vi "Noyito10ChannelADC_ManualPollingExample.vi"(8 "error in (no error)":errorcluster) -> (0 "error out":errorcluster, 1 "userMessage":string, 3 "readBuffer":string)   [LabVIEW 2020]
uses:
  <vilib>/Instr/_visa.llb/VISA Configure Serial Port (Instr).vi
panel:
  in  "Polling Speed":bool
  out "Num bytes":u32=115200
  in  "STOP POLLING":bool
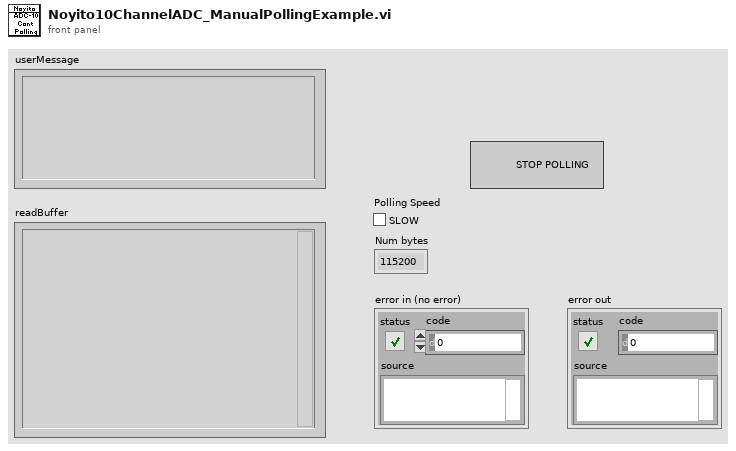
[diagram p1: front panel]
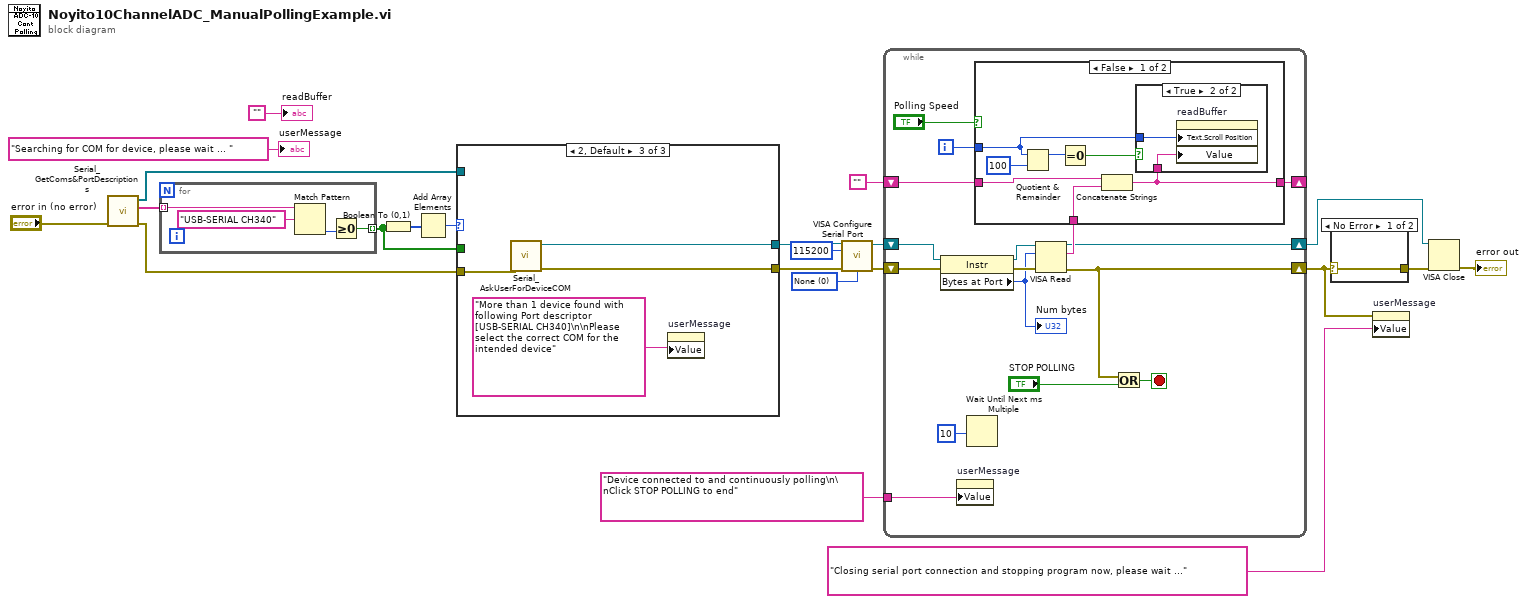
[diagram p0: block diagram]
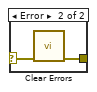
[diagram p2: hidden frame]
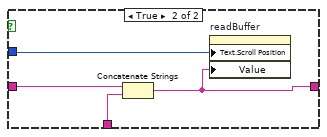
[diagram p4: hidden frame]
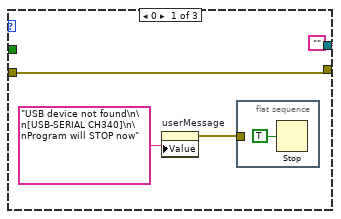
[diagram p5: hidden frame]
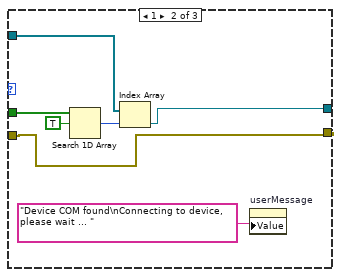
[diagram p6: hidden frame]
diagram:
  w11 = u16 0 items=["None", "XON/XOFF", "RTS/CTS", "XON/XOFF & RTS/CTS", "DTR/DSR", "XON/XOFF & DTR/DSR"] ("flow control (0:none)")
  n1 = call "Serial_GetComs&PortDescriptions.vi"("error in (no error)"="error in (no error)") -> ("error out"=w17:errorcluster, "WinsDescriptions"=w21:string[], "COMs"=w15:refnum<visa-resource-name>[])  [unwired: 8 in]
  n2 = for {
    tunnel: w21 -> [w26] mode=indexing
    tunnel: [w23] -> w16 mode=indexing
    n3 = Match Pattern(string=w26, regular expression="USB-SERIAL CH340") -> (offset past match=w24:i32)  [unwired: 1 in, 3 out]
    n4 = Greater Or Equal To 0?(x=w24) -> (x >= 0?=w23:bool)
  }
  n5 = Boolean To (0,1)(Boolean=w16) -> (0, 1=w20:i16[])
  n6 = Add Array Elements(numeric array=w20) -> (sum=w19:i16)
  n7 = case shown="2, Default" w19 {
    tunnel: w17 -> [w28 w32 w41]
    tunnel: [w28 w32 w40] -> w14
    tunnel: ["" w33 w39] -> w13
    tunnel: w16 -> [_ w37 _]
    tunnel: w15 -> [_ w34 _]
    frame 0 {
      n8 = property on="userMessage" class="Str"("Value"="USB device not found\n\n[USB-SERIAL CH340]\n\nProgram will STOP now" ("regular expression")) -> (error out=w29:errorcluster)  [unwired: 2 in, 1 out]
      n9 = flat-sequence {
        tunnel: w29 -> [_]
        frame #0 {
          n10 = Stop(stop? (T)=TRUE) -> ()
        }
      }
    }
    frame 1 {
      n11 = Search 1D Array(1D array=w37, element=TRUE) -> (index of element=w35:i32)  [unwired: 1 in]
      n12 = Index Array(array=w34, index=w35) -> (element=w33:refnum<visa-resource-name>)
      n13 = property on="userMessage" class="Str"("Value"="Device COM found\nConnecting to device, please wait ... " ("regular expression")) -> ()  [unwired: 2 in, 2 out]
    }
    frame 2, Default {
      n14 = call "Serial_AskUserForDeviceCOM.vi"("error in (no error)"=w41) -> ("error out"=w40:errorcluster, "Com-Out"=w39:refnum<visa-resource-name>)  [unwired: 9 in]
      n15 = property on="userMessage" class="Str"("Value"="More than 1 device found with following Port descriptor [USB-SERIAL CH340]\n\nPlease select the correct COM for the intended device" ("regular expression")) -> ()  [unwired: 2 in, 2 out]
    }
  }
  n16 = call-poly "VISA Configure Serial Port"("VISA resource name"=w13, "baud rate (9600)"=u32 115200, "error in (no error)"=w14, "flow control (0:none)"=w11) -> ("VISA resource name out"=w2:refnum<visa-resource-name>, "error out"=w1:errorcluster)  [unwired: 10 in]
  n17 = while {
    shift-right: [w48] -> w4
    shift-left: w1 -> [w46]
    shift-right: [w49] -> w9
    shift-left: w2 -> [w58]
    shift-right: [w44] -> _
    shift-left: "" -> [w52]
    tunnel: "Device connected to and continuously polling\n\nClick STOP POLLING to end" ("regular expression") -> [w51]
    i -> [w45]
    stop <- w54 stop-if-true
    n18 = property class="Instr"(reference=w58, error in=w46) -> (reference out=w56:refnum<visa-resource-name>, error out=w57:errorcluster, "Bytes at Port"=w50:u32)
    "Num bytes" <- w50
    n19 = property on="userMessage" class="Str"("Value"=w51) -> ()  [unwired: 2 in, 2 out]
    n20 = Wait Until Next ms Multiple(millisecond multiple=u32 10) -> ()  [unwired: 1 out]
    n21 = VISA Read(VISA resource name=w56, byte count=w50, error in (no error)=w57) -> (VISA resource name out=w49:refnum<visa-resource-name>, read buffer=w53:string, error out=w48:errorcluster)  [unwired: 1 out]
    n22 = case shown="False" "Polling Speed" {
      tunnel: w53 -> [w65 w71]
      tunnel: w52 -> [w64 w70]
      tunnel: [w61 w68] -> w44
      tunnel: w45 -> [w60 w69]
      frame False {
        n23 = Quotient & Remainder(x=w60, y=100) -> (x-y*floor(x/y)=w62:i32)  [unwired: 1 out]
        n24 = Equal To 0?(x=w62) -> (x = 0?=w59:bool)
        n25 = Concatenate Strings(w64, w65) -> (w61:string)
        n26 = case shown="True" w59 {
          tunnel: w61 -> [_ w67]
          tunnel: w60 -> [_ w66]
          frame False {
          }
          frame True {
            n27 = property on="readBuffer" class="Str"("Text.Scroll Position"=w66, "Value"=w67) -> ()  [unwired: 2 in, 2 out]
          }
        }
      }
      frame True {
        n28 = Concatenate Strings(w70, w71) -> (w68:string)
        n29 = property on="readBuffer" class="Str"("Text.Scroll Position"=w69, "Value"=w68) -> ()  [unwired: 2 in, 2 out]
      }
    }
    n30 = Or(x=w48, y="STOP POLLING") -> (x .or. y?=w54:bool)
  }
  n31 = case shown="No Error" w4 {
    selector: w4 -> [w72 w74]
    tunnel: [w72 w73] -> w10
    frame No Error {
    }
    frame Error {
      n32 = call <vilib>:"Clear Errors.vi"("error in (no error)"=w74) -> ("error out"=w73:errorcluster)  [unwired: 5 in, 1 out]
    }
  }
  n33 = property on="userMessage" class="Str"(error in=w4, "Value"="Closing serial port connection and stopping program now, please wait ..." ("regular expression")) -> ()  [unwired: 1 in, 2 out]
  n34 = VISA Close(VISA resource name=w9, error in (no error)=w10) -> (error out=→"error out":errorcluster)
  "userMessage" <- "Searching for COM for device, please wait ... " ("regular expression")
  "readBuffer" <- ""
